vi "generate_error.vi"(6 "show_call_chain":bool=TRUE, 8 "error in (no error)":errorcluster, 10 "data":variant, 11 "error":T1) -> (0 "error out":errorcluster)   [LabVIEW 2015, in "lv-bin.lvlib"]
uses:
  lv-bin.lvlib
  _controls/error.ctl
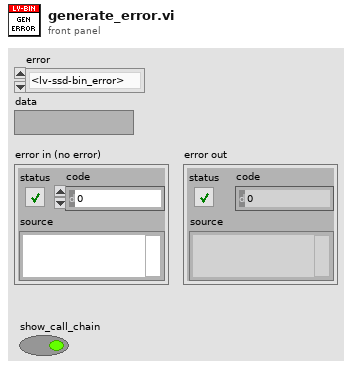
[diagram p1: front panel]
types:
  T1 = typedef "lv-bin.lvlib/error.ctl" = enum16{"<lv-ssd-bin_error>", "invalid_bad_path", "<null>"}
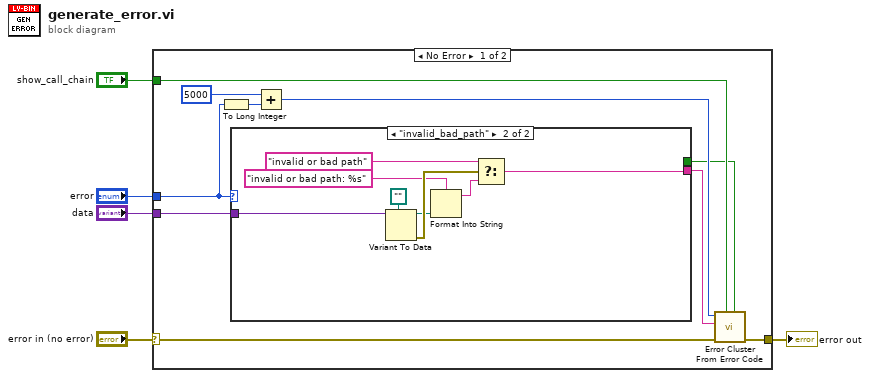
[diagram p0: block diagram]
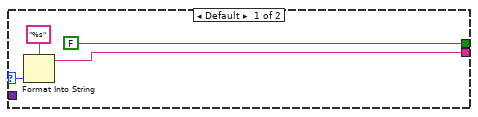
[diagram p2: hidden frame]
diagram:
  n1 = case shown="No Error" "error in (no error)" {
    selector: "error in (no error)" -> [w6 w28]
    tunnel: "data" -> [w15 _]
    tunnel: [w14 w28] -> w3
    tunnel: "error" -> [w12 _]
    tunnel: "show_call_chain" -> [w8 _]
    frame No Error {
      n2 = To Long Integer(number=w12) -> (32bit integer=w11:i32)
      n3 = case shown="\"invalid_bad_path\"" w12 {
        selector: w12 -> [w18 _]
        tunnel: w15 -> [_ w26]
        tunnel: [w17 w21] -> w9
        tunnel: [FALSE _] -> w7
        frame Default {
          n4 = Format Into String(format string="%s", w18) -> (resulting string=w17:string)  [unwired: 2 in, 1 out]
        }
        frame "invalid_bad_path" {
          n5 = Variant To Data(type=path "", Variant=w26) -> (data=w20:path, error out=w27:errorcluster)  [unwired: 1 in]
          n6 = Format Into String(format string="invalid or bad path: %s", w20) -> (resulting string=w22:string)  [unwired: 2 in, 1 out]
          n7 = Select(t="invalid or bad path" ("format string"), s=w27, f=w22) -> (s? t:f=w21:string)
        }
      }
      n8 = Add(x=5000, y=w11) -> (x+y=w10:i32)
      n9 = call <vilib>:"Error Cluster From Error Code.vi"("is warning? (False)"=w7, "show call chain? (False)"=w8, "error in (no error)"=w6, "error message (\"\")"=w9, "error code (0)"=w10) -> ("error out"=w14:errorcluster)  [unwired: 4 in]
    }
    frame Error {
    }
  }
  "error out" <- w3
